vi "EMV Check For Decreasing Temperatures.vi"(6 "Detect Flow Start?":bool, 8 "error in (no error)":errorcluster, 11 "Current T7 Temperatures":dbl[](array[numeric])) -> (0 "error out":errorcluster, 2 "Slope History":dbl[](array[numeric]), 3 "Current T7 Temperatures Output":dbl[](array[numeric]), 5 "Array Has a Slope":bool)   [LabVIEW 2016]
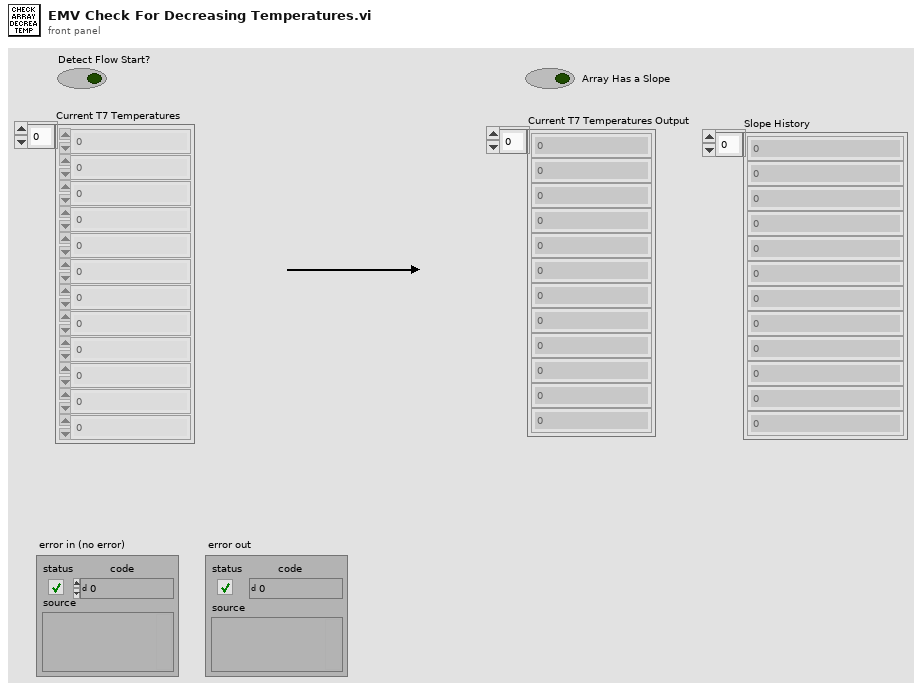
[diagram p1: front panel]
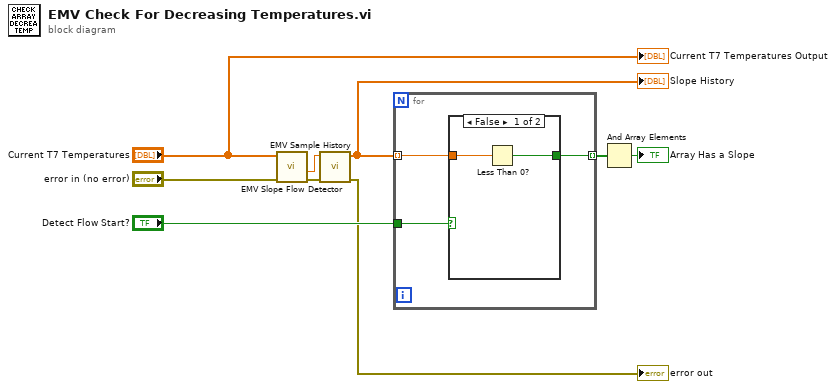
[diagram p0: block diagram]
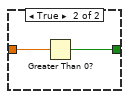
[diagram p2: hidden frame]
diagram:
  n1 = call "EMV Slope Flow Detector.vi"("error in (no error)"="error in (no error)", "Current T6 Temperatures in"="Current T7 Temperatures") -> ("error out"=w5:errorcluster, "slope"=w4:dbl)  [unwired: 5 in, 3 out]
  n2 = call "EMV Sample History.vi"("error in (no error)"=w5, "T6 Temp"=w4) -> ("error out"=→"error out":errorcluster, "T6 History"=w6:dbl[])  [unwired: 8 in]
  "Slope History" <- w6
  n3 = for {
    tunnel: w6 -> [w12] mode=indexing
    tunnel: [w11] -> w7 mode=indexing
    tunnel: "Detect Flow Start?" -> [w10]
    n4 = case shown="False" w10 {
      tunnel: w12 -> [w14 w16]
      tunnel: [w13 w15] -> w11
      frame False {
        n5 = Less Than 0?(x=w14) -> (x < 0?=w13:bool)
      }
      frame True {
        n6 = Greater Than 0?(x=w16) -> (x > 0?=w15:bool)
      }
    }
  }
  n7 = And Array Elements(Boolean array=w7) -> (logical AND=→"Array Has a Slope":bool)
  "Current T7 Temperatures Output" <- "Current T7 Temperatures"
